vi "Test File Info MP3.vi"(8 "error in (no error)":errorcluster) -> (0 "error out":errorcluster, 3 "Pass?":bool)   [LabVIEW 2020]
uses:
  G-Audio/Controls/Audio File Codec.ctl
  G-Audio/Controls/Audio File Info.ctl
  G-Audio/Audio Files/Polymorphic VIs/Get Audio File Info (Path).vi
  G-Audio/Private/Path To UTF-8 String.vi
  G-Audio/Audio Files/Private/Get Audio File Info (Core).vi
  G-Audio/Private/Result To Error.vi
  <vilib>/Utility/error.llb/Error Cluster From Error Code.vi
  G-Audio/G-Audio.lvlib
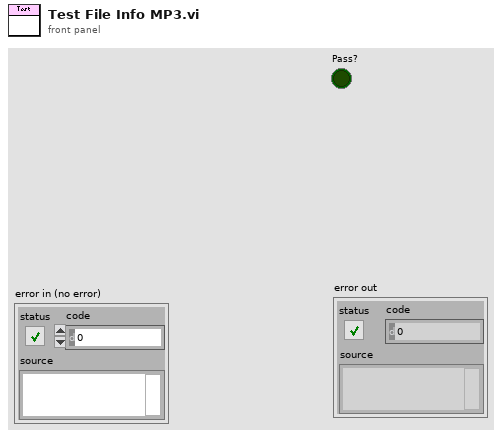
[diagram p1: front panel]
types:
  T1 = typedef "G-Audio.lvlib/Audio File Info.ctl" = cluster{"Sample Rate (Hz)":u32, "Channels":u32, "Bit Depth":u32}
  T2 = typedef "G-Audio.lvlib/Audio File Codec.ctl" = enum16{"flac", "mp3", "vorbis", "wav", "unsupported"}
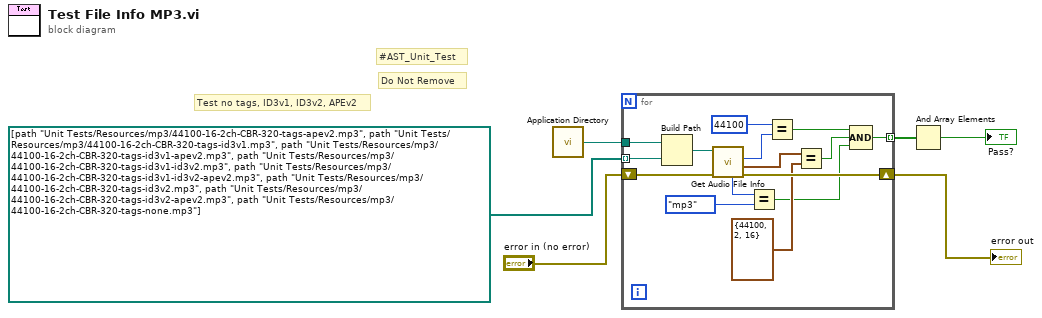
[diagram p0: block diagram]
diagram:
  # "Test no tags, ID3v1, ID3v2, APEv2"
  # "Do Not Remove"
  # "#AST_Unit_Test"
  n1 = call <vilib>:"Application Directory.vi"() -> ("Application Directory"=w5:path)
  n2 = for {
    tunnel: w5 -> [w21]
    shift-right: [w19] -> w1
    shift-left: "error in (no error)" -> [w18]
    tunnel: path[] [path "Unit Tests/Resources/mp3/44100-16-2ch-CBR-320-tags-apev2.mp3", path "Unit Tests/Resources/mp3/44100-16-2ch-CBR-320-tags-id3v1.mp3", path "Unit Tests/Resources/mp3/44100-16-2ch-CBR-320-tags-id3v1-apev2.mp3", path "Unit Tests/Resources/mp3/44100-16-2ch-CBR-320-tags-id3v1-id3v2.mp3", path "Unit Tests/Resources/mp3/44100-16-2ch-CBR-320-tags-id3v1-id3v2-apev2.mp3", path "Unit Tests/Resources/mp3/44100-16-2ch-CBR-320-tags-id3v2.mp3", path "Unit Tests/Resources/mp3/44100-16-2ch-CBR-320-tags-id3v2-apev2.mp3", path "Unit Tests/Resources/mp3/44100-16-2ch-CBR-320-tags-none.mp3"] -> [w17] mode=indexing
    tunnel: [w7] -> w2 mode=indexing
    n3 = Build Path(base path=w21, name or relative path=w17) -> (appended path=w20:path)
    n4 = call-poly "Get Audio File Info.vi"("error in (no error)"=w18, "Path In"=w20) -> ("error out"=w19:errorcluster, "Audio File Info"=w12:T1, "PCM Frame Length"=w14:u64, "Codec"=w16:T2)  [unwired: 5 in, 1 out]
    n5 = Equal?(x=w16, y=Audio_File_Codec."mp3" ("x")) -> (x = y?=w10:bool)
    n6 = Equal?(x=u64 44100, y=w14) -> (x = y?=w8:bool)
    n7 = Equal?(x=w12, y=T1 {"Sample Rate (Hz)"=44100, "Channels"=2, "Bit Depth"=16} ("Audio File Info")) -> (x = y?=w9:bool)
    n8 = Compound Arithmetic op=AND(w8, w9, w10) -> (w7:bool)
  }
  "error out" <- w1
  n9 = And Array Elements(Boolean array=w2) -> (logical AND=→"Pass?":bool)
